vi "AO Update Channel.vi"   [LabVIEW 2009]
doc: "Writes a specified value to an analog output channel."
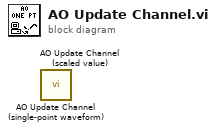
[diagram p0: block diagram]
diagram:
  n1 = call "AO Update Channel (single-point waveform).vi"() -> ()  [unwired: 3 in]
  n2 = call "AO Update Channel (scaled value).vi"() -> ()  [unwired: 3 in]
